vi "Facade_RCM.vi"(0 "Data In":T4, 2 "Display State In":T2={"RCM File Path"=path "", "Left"=0, "Top"=0, "Font Name"="", "Font Size"=-26986, "Font Color"=26367, "Separator Color"=9868950, "Frame Color"=9868950, "Overlay Color"=26367}, 3 "Container State":T3) -> (6 "Data Out":T4, 7 "Display State Out":T2={"RCM File Path"=path "", "Left"=0, "Top"=0, "Font Name"="", "Font Size"=-26986, "Font Color"=26367, "Separator Color"=9868950, "Frame Color"=9868950, "Overlay Color"=26367}, 8 "Action":T1)   [LabVIEW 2009, in "RCM.xctl"]
uses:
  RCM.xctl
  Data_RCM.ctl
  <vilib>/_xctls/Container State.ctl
  State_RCM.ctl
  <vilib>/_xctls/Action.ctl
  <vilib>/_xctls/XControlSupport.lvlib
panel:
  # "This is the Right Click Menu XControl.\nHide this control when you run your application.\nYou can launch RCM Editor by right clicking this xcontrol."
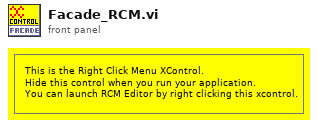
[diagram p1: front panel]
types:
  T1 = typedef "XControlSupport.lvlib/Action.ctl" = cluster{"Data Changed?":bool, "State Changed?":bool, "Action Name":string}
  T2 = typedef "RCM.xctl/State_RCM.ctl" = cluster{"RCM File Path":path, "Left":u32, "Top":u32, "Font Name":string, "Font Size":i16, "Font Color":u32, "Separator Color":u32, "Frame Color":u32, "Overlay Color":u32}
  T3 = typedef "XControlSupport.lvlib/Container State.ctl" = cluster{"Indicator?":bool, "Run Mode?":bool, " Refnum":refnum<vi>}
  T4 = typedef "RCM.xctl/Data_RCM.ctl" = string
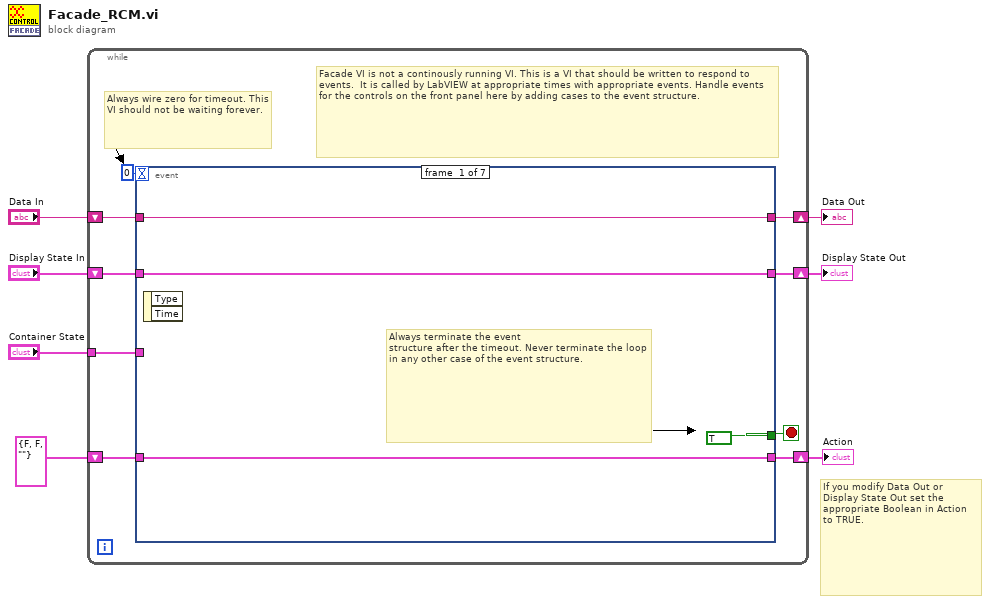
[diagram p0: block diagram]
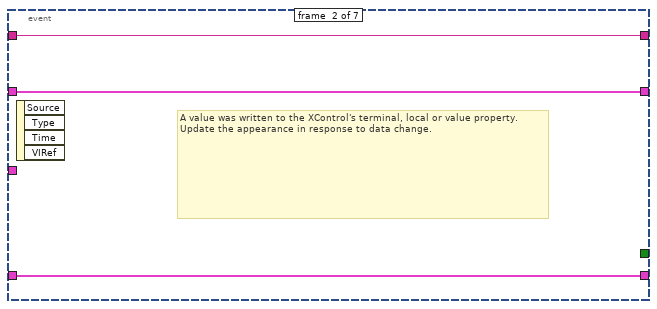
[diagram p2: hidden frame]
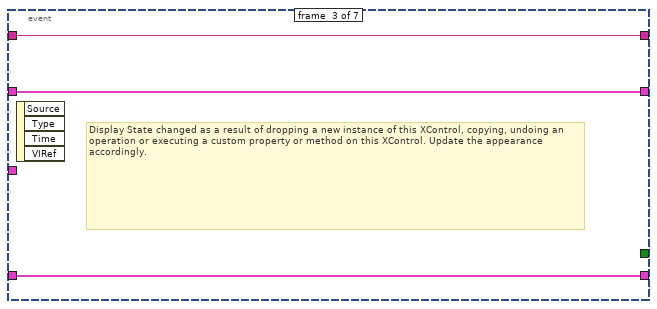
[diagram p3: hidden frame]
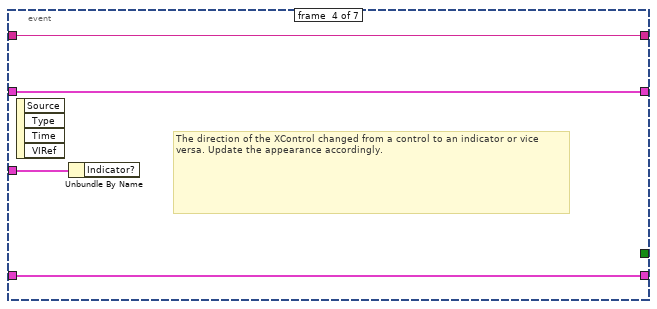
[diagram p4: hidden frame]
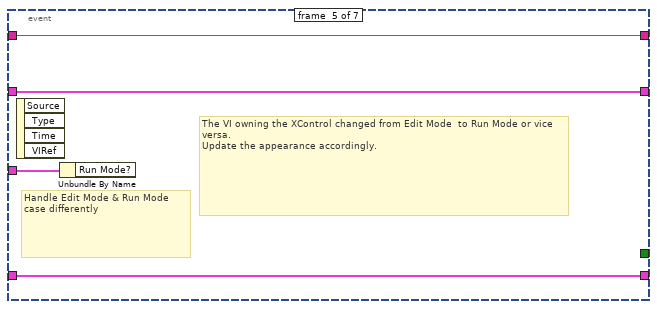
[diagram p5: hidden frame]
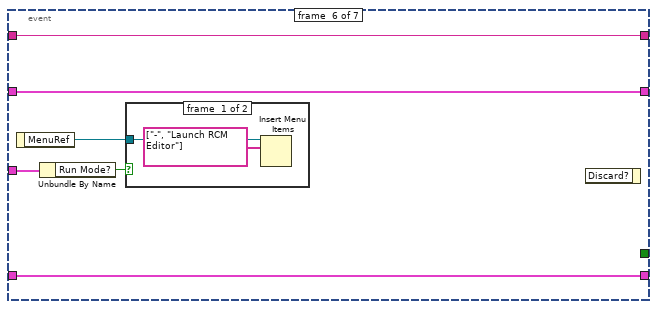
[diagram p6: hidden frame]
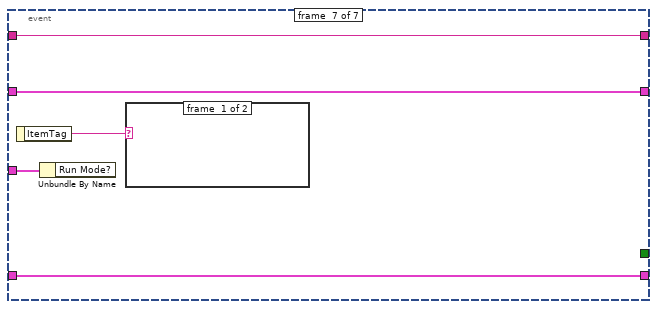
[diagram p8: hidden frame]
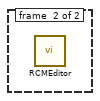
[diagram p9: hidden frame]
diagram:
  # "If you modify Data Out or\nDisplay State Out set the\nappropriate Boolean in Action\nto TRUE."
  n1 = while {
    shift-right: [w15] -> w4
    shift-left: "Display State In" -> [w16]
    tunnel: "Container State" -> [w12]
    shift-right: [w10] -> w7
    shift-left: "Data In" -> [w11]
    shift-right: [w8] -> w2
    shift-left: T1 {"Data Changed?"=FALSE, "State Changed?"=FALSE, "Action Name"=""} ("Action") -> [w9]
    stop <- w14 stop-if-true
    # "Facade VI is not a continously running VI. This is a VI that should be written to respond to events.  It is called by LabVIEW at appropriate times with appropriate events. Handle events for the controls on the front panel here by adding cases to the event structure."
    # "Always wire zero for timeout. This\nVI should not be waiting forever."
    n2 = event shown="[5] \"Pane\": Shortcut Menu Activation?" {
      selector: _ -> [_ _ _ _ _ _ _]
      dyn-events: _ -> [_ _ _ _ _ _ _]
      timeout: 0 -> [_ _ _ _ _ _ _]
      tunnel: w16 -> [w18 w22 w26 w29 w33 w40 w47]
      tunnel: [w18 w22 w26 w29 w33 w40 w47] -> w15
      tunnel: [TRUE _ _ _ _ _ _] -> w14
      tunnel: w12 -> [_ _ _ w30 w34 w37 w44]
      tunnel: w11 -> [w17 w23 w25 w28 w32 w39 w46]
      tunnel: [w17 w23 w25 w28 w32 w39 w46] -> w10
      tunnel: [w19 w21 w24 w27 w31 w38 w45] -> w8
      tunnel: w9 -> [w19 w21 w24 w27 w31 w38 w45]
      event #0 {
        # "Always terminate the event\nstructure after the timeout. Never terminate the loop in any other case of the event structure."
        n3 = event-data() -> ()  [unwired: 1 in, 2 out]
      }
      event #1 {
        # "A value was written to the XControl's terminal, local or value property.\nUpdate the appearance in response to data change."
        n4 = event-data() -> ()  [unwired: 1 in, 4 out]
      }
      event #2 {
        # "Display State changed as a result of dropping a new instance of this XControl, copying, undoing an operation or executing a custom property or method on this XControl. Update the appearance accordingly."
        n5 = event-data() -> ()  [unwired: 1 in, 4 out]
      }
      event #3 {
        # "The direction of the XControl changed from a control to an indicator or vice versa. Update the appearance accordingly."
        n6 = event-data() -> ()  [unwired: 1 in, 4 out]
        n7 = Unbundle By Name(w30) -> ()  [unwired: 1 out]
      }
      event #4 {
        # "The VI owning the XControl changed from Edit Mode  to Run Mode or vice versa.\nUpdate the appearance accordingly."
        # "Handle Edit Mode & Run Mode\ncase differently"
        n8 = event-data() -> ()  [unwired: 1 in, 4 out]
        n9 = Unbundle By Name(w34) -> ()  [unwired: 1 out]
      }
      event #5 {
        n10 = event-data() -> ("MenuRef"=w35:refnum<k9>)  [unwired: 1 in]
        n11 = Unbundle By Name(w37) -> ("Run Mode?"=w36:bool)
        n12 = case shown="False" w36 {
          tunnel: w35 -> [w42 _]
          frame #0 {
            n13 = Insert Menu Items(8:string[] ["-", "Launch RCM Editor"] ("item names"), 9:w42) -> ()  [unwired: 4 in, 3 out]
          }
          frame #1 {
          }
        }
        n14 = event-data() -> ()  [unwired: 2 in, 1 out]
      }
      event #6 {
        n15 = event-data() -> ("ItemTag"=w43:string)  [unwired: 1 in]
        n16 = Unbundle By Name(w44) -> ()  [unwired: 1 out]
        n17 = case shown="\"Launch RCM Editor\"" w43 {
          frame #0 {
          }
          frame #1 {
            n18 = call "RCMEditor.vi"() -> ()  [unwired: 1 in]
          }
        }
      }
    }
  }
  "Display State Out" <- w4
  "Data Out" <- w7
  "Action" <- w2
